vi "LS4 SetLimit_SD.vi"(1 "MaxRange":dbl format="%.2f", 2 "MinRange":dbl format="%.2f", 3 "Axis":i32=1) -> (0 "Command executed":bool)   [LabVIEW 2015]
uses:
  DLL/LStep4.dll
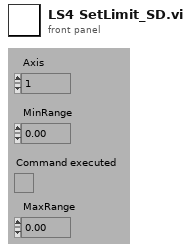
[diagram p1: front panel]
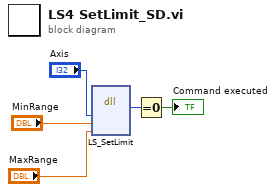
[diagram p0: block diagram]
diagram:
  n1 = dll-call lib="G:/SD/TRANCON/DLL/LStep4.dll" fn="LS_SetLimit"("Axis"="Axis", "MinRange"="MinRange", "MaxRange"="MaxRange") -> ("type de retour"=w5:i32)  [unwired: 6 in, 2 out]
  n2 = Equal To 0?(x=w5) -> (x = 0?=→"Command executed":bool)
